vi "Triax320 Initialize.vi"() -> ()   [LabVIEW 2019]
uses:
  <userlib>/Triax320/Triax Init States.ctl
panel:
  out "ChaineRep":string caption="Chaîne de réponse"
  in  "Triax VISA Rsrc":refnum<visa-resource-name>="SR530"
  out "error out":errorcluster
  in  "error in (no error)":errorcluster
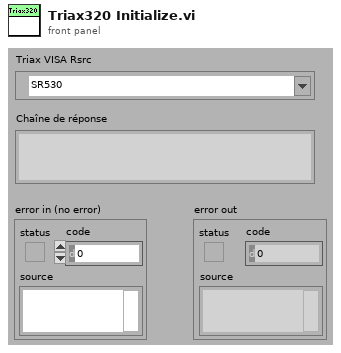
[diagram p1: front panel]
types:
  T1 = typedef "Triax Init States.ctl" = enum16{"CheckMode", "Reboot", "MainProg", "Set Int Mode", "init"}
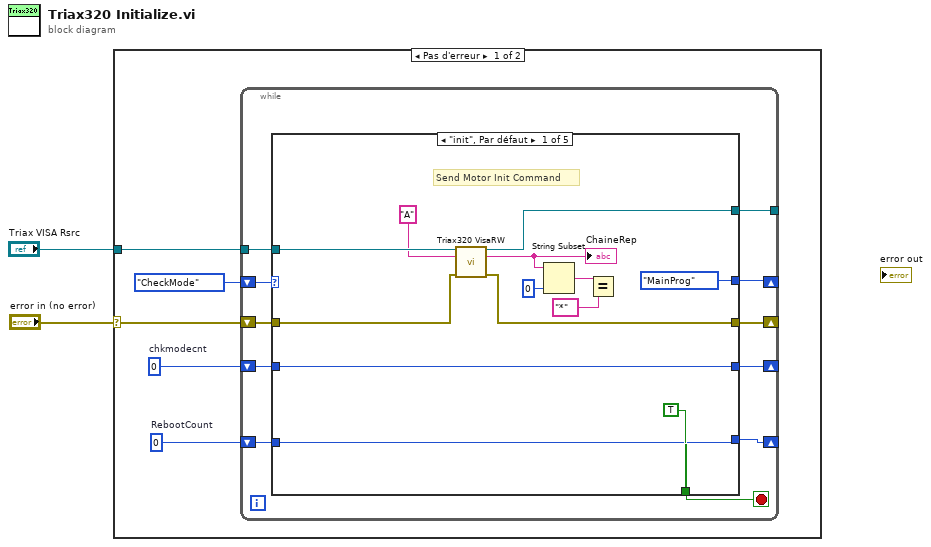
[diagram p0: block diagram]
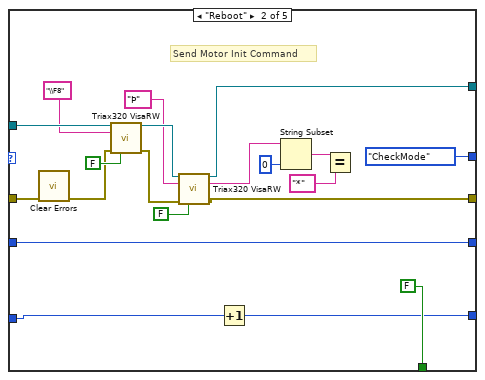
[diagram p2: hidden frame]
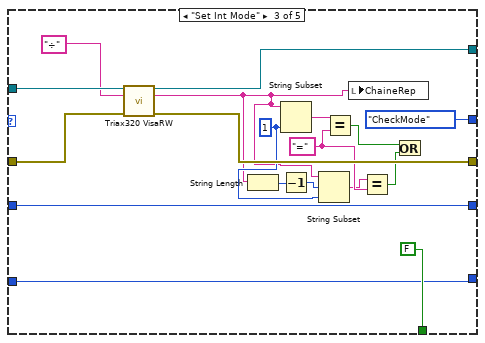
[diagram p3: hidden frame]
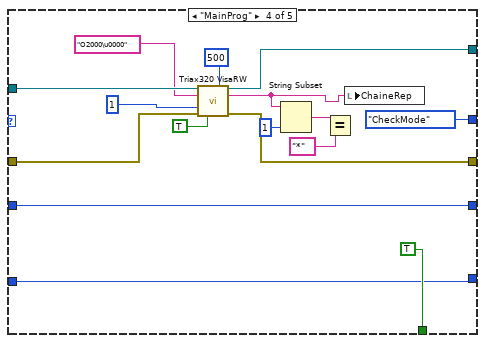
[diagram p4: hidden frame]
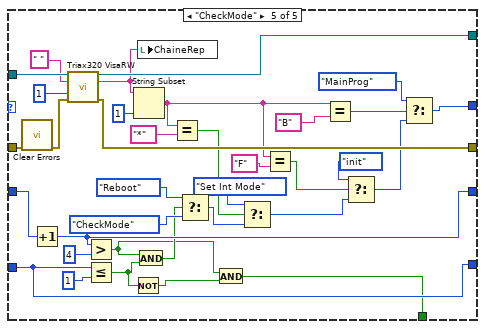
[diagram p5: hidden frame]
diagram:
  n1 = case shown="Pas d'erreur" "error in (no error)" {
    selector: "error in (no error)" -> [w5 _]
    tunnel: "Triax VISA Rsrc" -> [w6 _]
    frame No Error {
      w3 = 0  # RebootCount
      w4 = 0  # chkmodecnt
      n2 = while {
        shift-right: [w16] -> _
        shift-left: Triax_Init_States."CheckMode" ("Triax Init States") -> [w18]
        tunnel: w6 -> [w15]
        shift-right: [w13] -> _
        shift-left: w5 -> [w14]
        tunnel: [w12] -> _
        shift-right: [w11] -> _
        shift-left: w4 -> [w10]
        shift-right: [w8] -> _
        shift-left: w3 -> [w9]
        stop <- w17 stop-if-true
        n3 = case shown="\"init\", Par défaut" w18 {
          tunnel: [TRUE FALSE FALSE TRUE w88] -> w17
          tunnel: [Triax_Init_States."MainProg" ("Triax Init States") Triax_Init_States."CheckMode" ("Triax Init States") Triax_Init_States."CheckMode" ("Triax Init States") Triax_Init_States."CheckMode" ("Triax Init States") w107] -> w16
          tunnel: w15 -> [w29 w49 w67 w83 w120]
          tunnel: w14 -> [w28 w48 w66 w82 w119]
          tunnel: [w27 w37 w65 w81 w118] -> w13
          tunnel: [w25 w38 w64 w80 w117] -> w12
          tunnel: [w20 w35 w61 w71 w95] -> w11
          tunnel: w10 -> [w20 w35 w61 w71 w100]
          tunnel: w9 -> [w19 w34 w60 w70 w92]
          tunnel: [w19 w33 w60 w70 w92] -> w8
          frame "init", Default {
            # "Send Motor Init Command"
            n4 = call <userlib>:"Triax320 VisaRW.vi"("VISA Rsrc"=w29, "ChaineCom"="A", "error in (no error)"=w28) -> ("VISA Rsrc Out"=w25:refnum<visa-resource-name>, "ChaineRep"=w24:string, "error out"=w27:errorcluster)  [unwired: 7 in, 3 out]
            "ChaineRep" <- w24
            n5 = String Subset(string=w24, length (rest)=0 ("longueur (reste)")) -> (substring=w22:string)  [unwired: 1 in]
            n6 = Equal?(x=w22, y="*") -> ()  [unwired: 1 out]
          }
          frame "Reboot" {
            # "Send Motor Init Command"
            n7 = call <vilib>:"Clear Errors.vi"("error in (no error)"=w48) -> ("error out"=w32:errorcluster)  [unwired: 5 in, 1 out]
            n8 = call <userlib>:"Triax320 VisaRW.vi"("VISA Rsrc"=w49, "ChaineCom"="\\F8", "error in (no error)"=w32, "Lecture?(T)"=FALSE) -> ("VISA Rsrc Out"=w42:refnum<visa-resource-name>, "error out"=w43:errorcluster)  [unwired: 6 in, 4 out]
            n9 = call <userlib>:"Triax320 VisaRW.vi"("VISA Rsrc"=w42, "ChaineCom"="Þ", "error in (no error)"=w43, "Lecture?(T)"=FALSE) -> ("VISA Rsrc Out"=w38:refnum<visa-resource-name>, "ChaineRep"=w36:string, "error out"=w37:errorcluster)  [unwired: 6 in, 3 out]
            n10 = Increment(x=w34) -> (x+1=w33:i32)
            n11 = String Subset(string=w36, length (rest)=0 ("longueur (reste)")) -> (substring=w45:string)  [unwired: 1 in]
            n12 = Equal?(x=w45, y="*") -> ()  [unwired: 1 out]
          }
          frame "Set Int Mode" {
            w56 = "=" ("y")
            w57 = 1 ("longueur (reste)")
            n13 = call <userlib>:"Triax320 VisaRW.vi"("VISA Rsrc"=w67, "ChaineCom"="÷" ("chaîne"), "error in (no error)"=w66) -> ("VISA Rsrc Out"=w64:refnum<visa-resource-name>, "ChaineRep"=w54:string, "error out"=w65:errorcluster)  [unwired: 7 in, 3 out]
            n14 = String Length(string=w54) -> (length=w59:i32)
            n15 = String Subset(string=w54, length (rest)=w57) -> (substring=w63:string)  [unwired: 1 in]
            n16 = Decrement(x=w59) -> (x-1=w58:i32)
            n17 = String Subset(string=w54, offset (0)=w58, length (rest)=w57) -> (substring=w55:string)
            n18 = Equal?(x=w63, y=w56) -> (x = y?=w53:bool)
            n19 = local write "ChaineRep"(w54) -> ()
            n20 = Equal?(x=w55, y=w56) -> (x = y?=w52:bool)
            n21 = Or(x=w53, y=w52) -> ()  [unwired: 1 out]
          }
          frame "MainProg" {
            n22 = call <userlib>:"Triax320 VisaRW.vi"("VISA Rsrc"=w83, "Délais (0 ms)"=u32 500, "ChaineCom"="O2000\u0000" ("chaîne"), "Nbcaract"=u32 1, "error in (no error)"=w82, "Lecture?(T)"=TRUE) -> ("VISA Rsrc Out"=w80:refnum<visa-resource-name>, "ChaineRep"=w72:string, "error out"=w81:errorcluster)  [unwired: 4 in, 3 out]
            n23 = String Subset(string=w72, length (rest)=1 ("longueur (reste)")) -> (substring=w78:string)  [unwired: 1 in]
            n24 = Equal?(x=w78, y="*") -> ()  [unwired: 1 out]
            n25 = local write "ChaineRep"(w72) -> ()
          }
          frame "CheckMode" {
            n26 = call <vilib>:"Clear Errors.vi"("error in (no error)"=w119) -> ("error out"=w87:errorcluster)  [unwired: 5 in, 1 out]
            n27 = Increment(x=w100) -> (x+1=w95:i32)
            n28 = call <userlib>:"Triax320 VisaRW.vi"("VISA Rsrc"=w120, "ChaineCom"=" " ("chaîne"), "Nbcaract"=u32 1, "error in (no error)"=w87) -> ("VISA Rsrc Out"=w117:refnum<visa-resource-name>, "ChaineRep"=w105:string, "error out"=w118:errorcluster)  [unwired: 6 in, 3 out]
            n29 = Greater?(x=w95, y=4) -> (0:w90:bool)
            n30 = Less Or Equal?(x=w92, y=1) -> (x <= y?=w89:bool)
            n31 = Not(x=w89) -> (.not. x?=w86:bool)
            n32 = String Subset(string=w105, length (rest)=1 ("longueur (reste)")) -> (substring=w97:string)  [unwired: 1 in]
            n33 = And(x=w90, y=w89) -> (x .and. y?=w91:bool)
            n34 = local write "ChaineRep"(w105) -> ()
            n35 = Equal?(x=w97, y="*") -> (x = y?=w104:bool)
            n36 = Select(t=Triax_Init_States."Reboot" ("Triax Init States"), s=w91, f=Triax_Init_States."CheckMode" ("Triax Init States")) -> (s? t:f=w93:T1)
            n37 = And(x=w90, y=w86) -> (x .and. y?=w88:bool)
            n38 = Select(t=Triax_Init_States."Set Int Mode" ("Triax Init States"), s=w104, f=w93) -> (s? t:f=w101:T1)
            n39 = Equal?(x=w97, y="F") -> (x = y?=w111:bool)
            n40 = Equal?(x=w97, y="B") -> (x = y?=w110:bool)
            n41 = Select(t=Triax_Init_States."init" ("Triax Init States"), s=w111, f=w101) -> (s? t:f=w109:T1)
            n42 = Select(t=Triax_Init_States."MainProg" ("Triax Init States"), s=w110, f=w109) -> (s? t:f=w107:T1)
          }
        }
      }
    }
    frame Error {
    }
  }
